vi "Create Clip Plane.vi"(5 "Type":enum16{"Max", "Min"}(ring), 7 "Axis":enum16{"X-Axis", "Y-Axis", "Z-Axis"}(ring), 8 "error in (no error)":errorcluster, 9 "Max":sgl, 10 "Min":sgl, 11 "Plot Object In":refnum<vi>) -> (0 "error out":errorcluster, 3 "Plot Object Out":refnum<vi>)   [LabVIEW 2020, in "3D Plot.lvclass"]
uses:
  <vilib>/Math Plots/3D Math Plots/3D Plot/3D Plot/3D Plot.lvclass
  <vilib>/picture/3D Picture Control/NI_3D Picture Control.lvlib
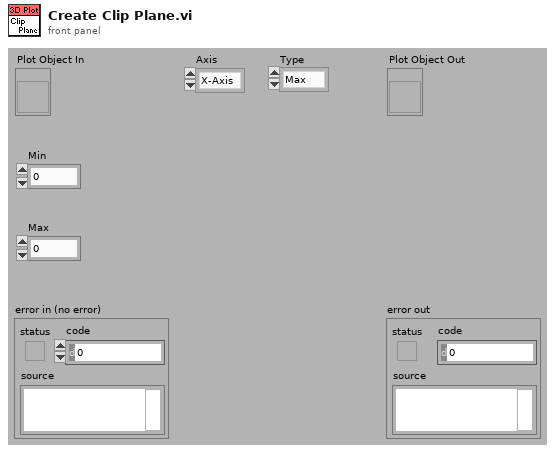
[diagram p1: front panel]
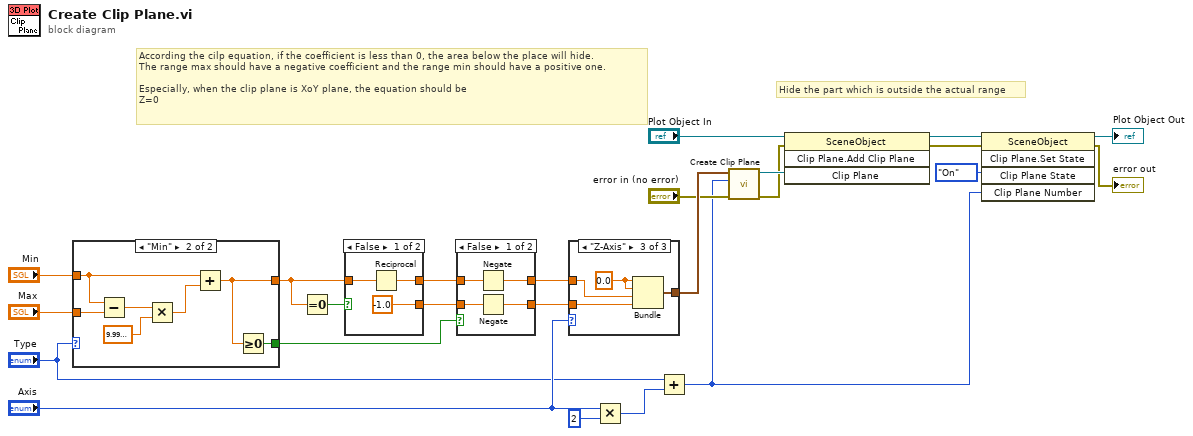
[diagram p0: block diagram]
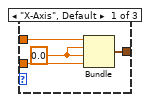
[diagram p2: hidden frame]
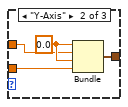
[diagram p3: hidden frame]
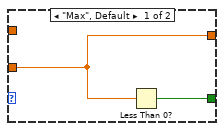
[diagram p4: hidden frame]
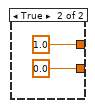
[diagram p6: hidden frame]
diagram:
  # "Hide the part which is outside the actual range"
  # "According the cilp equation, if the coefficient is less than 0, the area below the place will hide.\nThe range max should have a negative coefficient and the range min should have a positive one.\n\nEspecially, when the clip plane is XoY plane, the equation should be\nZ=0"
  n1 = case shown="\"Min\"" "Type" {
    tunnel: [w26 w28] -> w13
    tunnel: "Min" -> [_ w30]
    tunnel: "Max" -> [w26 w29]
    tunnel: [w25 w27] -> w6
    frame "Max", Default {
      n2 = Less Than 0?(x=w26) -> (x < 0?=w25:bool)
    }
    frame "Min" {
      n3 = Subtract(x=w30, y=w29) -> (x-y=w33:sgl)
      n4 = Multiply(x=w33, y=sgl 0.0001 ("X")) -> (x*y=w31:sgl)
      n5 = Add(x=w30, y=w31) -> (x+y=w28:sgl)
      n6 = Greater Or Equal To 0?(x=w28) -> (x >= 0?=w27:bool)
    }
  }
  n7 = Equal To 0?(x=w13) -> (x = 0?=w24:bool)
  n8 = case shown="False" w24 {
    tunnel: w13 -> [w35 _]
    tunnel: [w36 sgl 1.0 ("B")] -> w23
    tunnel: [sgl -1.0 sgl 0.0 ("B")] -> w22
    frame False {
      n9 = Reciprocal(x=w35) -> (1/x=w36:sgl)
    }
    frame True {
    }
  }
  n10 = case shown="False" w6 {
    tunnel: w23 -> [w39 w44]
    tunnel: [w40 w44] -> w8
    tunnel: w22 -> [w42 w43]
    tunnel: [w41 w43] -> w7
    frame False {
      n11 = Negate(x=w39) -> (-x=w40:sgl)
      n12 = Negate(x=w42) -> (-x=w41:sgl)
    }
    frame True {
    }
  }
  n13 = case shown="\"Z-Axis\"" "Axis" {
    tunnel: [w48 w49 w55] -> w19
    tunnel: w8 -> [w46 w51 w54]
    tunnel: w7 -> [w45 w50 w53]
    frame "X-Axis", Default {
      w47 = sgl 0.0 ("B")
      n14 = Bundle("B"=w46, "B"=w47, "B"=w47, "B"=w45) -> (w48:cluster{"B":sgl, "B":sgl, "B":sgl, "B":sgl})  [unwired: 1 out]
    }
    frame "Y-Axis" {
      w52 = sgl 0.0 ("B")
      n15 = Bundle("B"=w52, "B"=w51, "B"=w52, "B"=w50) -> (w49:cluster{"B":sgl, "B":sgl, "B":sgl, "B":sgl})  [unwired: 1 out]
    }
    frame "Z-Axis" {
      w56 = sgl 0.0 ("B")
      n16 = Bundle("B"=w56, "B"=w56, "B"=w54, "B"=w53) -> (w55:cluster{"B":sgl, "B":sgl, "B":sgl, "B":sgl})  [unwired: 1 out]
    }
  }
  n17 = Multiply(x="Axis", y=2) -> (x*y=w3:i32)
  n18 = Add(x="Type", y=w3) -> (x+y=w1:i32)
  n19 = call <vilib>:"Create Clip Plane.vi"("error in (no error)"="error in (no error)", "Number"=w1, "Plane"=w19) -> ("error out"=w15:errorcluster, "New Clip Plane Refnum"=w21:refnum<vi>)  [unwired: 7 out]
  n20 = invoke class="SceneObject" method="Clip Plane.Add Clip Plane"(reference="Plot Object In", error in=w15, "Clip Plane"=w21) -> (reference out=w18:refnum<vi>, error out=w17:errorcluster)  [unwired: 1 in, 2 out]
  n21 = invoke class="SceneObject" method="Clip Plane.Set State"(reference=w18, error in=w17, "Clip Plane State"=enum16{"Inherit Value", "Off", "On"}."On", "Clip Plane Number"=w1) -> (reference out=→"Plot Object Out":refnum<vi>, error out=→"error out":errorcluster)  [unwired: 1 in, 3 out]
